vi "Close All Current Shunts.vi"(8 "error in":errorcluster, 11 "Scan Configuration":T2[](array[typedef]) {"Resolution in Digits" items=["3 1/2"=3.5, "4 1/2"=4.5, "5 1/2"=5.5, "6 1/2"=6.5, "7 1/2"=7.5]}) -> (0 "error out":errorcluster, 3 "Array of Shunt to close":T1[](array[typedef]))   [LabVIEW 2021, in "DMM_Scan PXI RLY Driver 32V-16C.lvlib"]
doc: "Uses the scan configuration to return only the current channels and formats them in Individual Switch Relay format."
uses:
  DMM_Scan PXI RLY Driver 32V-16C.lvlib
  Typedefs/Scan configuration.ctl
  <instrlib>/niDMM/nidmm.llb/niDMM Resolution in Digits.ctl
  Static Digital Path Generation/Typedefs/Terminal and State Settings.ctl
  Static Digital Path Generation/Switch_Static Digital Path Generation.lvlib
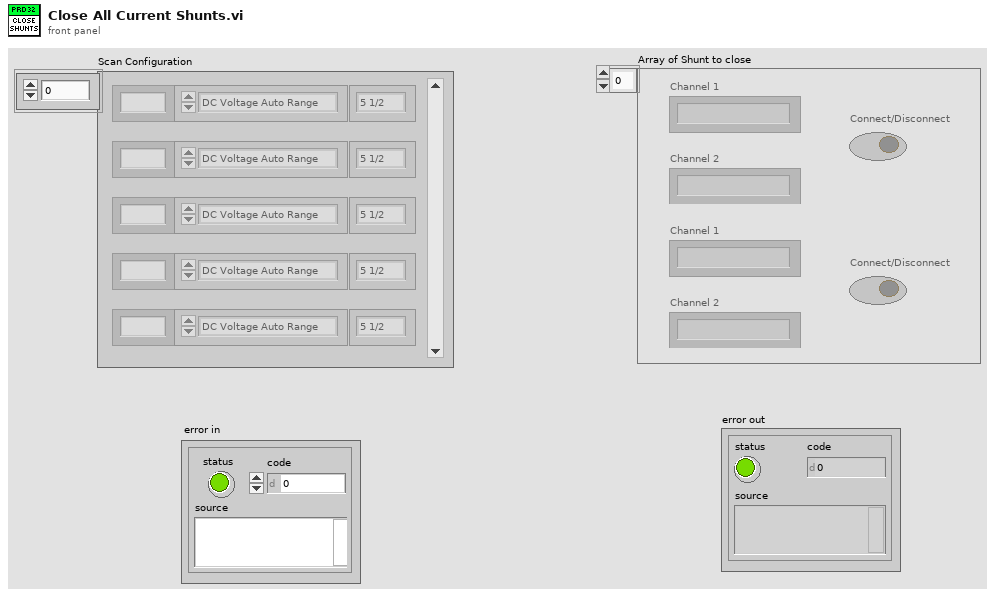
[diagram p1: front panel]
types:
  T1 = typedef "Switch_Static Digital Path Generation.lvlib/Terminal and State Settings.ctl" = cluster{"Connect/Disconnect":bool, "Channel 1":string, "Channel 2":string}
  T2 = typedef "DMM_Scan PXI RLY Driver 32V-16C.lvlib/Scan configuration.ctl" = cluster{"Channel":string, "Resolution in Digits":T3, "Range and Function":enum16{"DC Voltage Auto Range", "DC 100 mV", "DC 1 V ", "DC 10 V", "DC 100 V", "DC 300 V", " ", "AC Voltage Auto Range", "AC 50 mV", "AC 200 mV", "AC 500 mV", "AC 2 V", "AC 5 V", "AC 20 V", "AC 50 V", "AC 300 V", "  ", "DC Current Auto Range", "DC 1 uA", "DC 10 uA", "DC 100 uA", "DC 1 mA", "DC 10 mA", "DC 20 mA", "DC 100 mA", "DC 200 mA", "DC 1 A", "DC 3 A", "   ", "AC Current Auto Range", "AC 100 uA", "AC 1 mA", "AC 10 mA", "AC 100 mA", "AC 500 mA", "AC 1 A", "AC 3 A", "    ", "Resistance Auto Range", "Res 100 Ohm", "Res 1 kOhm", "Res 10 kOhm", "Res 100 kOhm", "Res 1 MOhm", "Res 10 MOhm", "Res 100 MOhm", "Res 5 GOhm", "     ", "Frequency AC Auto Range", "Freq AC 50 mV", "Freq AC 500 mV", "Freq AC 5 V", "Freq AC 50 V", "Freq AC 300 V", "      ", "Period AC Auto Range", "Period AC 50 mV", "Period AC 500 mV", "Period AC 5 V", "Period AC 50 V", "Period AC 300 V"}}
  T3 = typedef "niDMM Resolution in Digits.ctl" = dbl
  T4 = enum16{"DC Voltage Auto Range", "DC 100 mV", "DC 1 V ", "DC 10 V", "DC 100 V", "DC 300 V", " ", "AC Voltage Auto Range", "AC 50 mV", "AC 200 mV", "AC 500 mV", "AC 2 V", "AC 5 V", "AC 20 V", "AC 50 V", "AC 300 V", "  ", "DC Current Auto Range", "DC 1 uA", "DC 10 uA", "DC 100 uA", "DC 1 mA", "DC 10 mA", "DC 20 mA", "DC 100 mA", "DC 200 mA", "DC 1 A", "DC 3 A", "   ", "AC Current Auto Range", "AC 100 uA", "AC 1 mA", "AC 10 mA", "AC 100 mA", "AC 500 mA", "AC 1 A", "AC 3 A", "    ", "Resistance Auto Range", "Res 100 Ohm", "Res 1 kOhm", "Res 10 kOhm", "Res 100 kOhm", "Res 1 MOhm", "Res 10 MOhm", "Res 100 MOhm", "Res 5 GOhm", "     ", "Frequency AC Auto Range", "Freq AC 50 mV", "Freq AC 500 mV", "Freq AC 5 V", "Freq AC 50 V", "Freq AC 300 V", "      ", "Period AC Auto Range", "Period AC 50 mV", "Period AC 500 mV", "Period AC 5 V", "Period AC 50 V", "Period AC 300 V"}
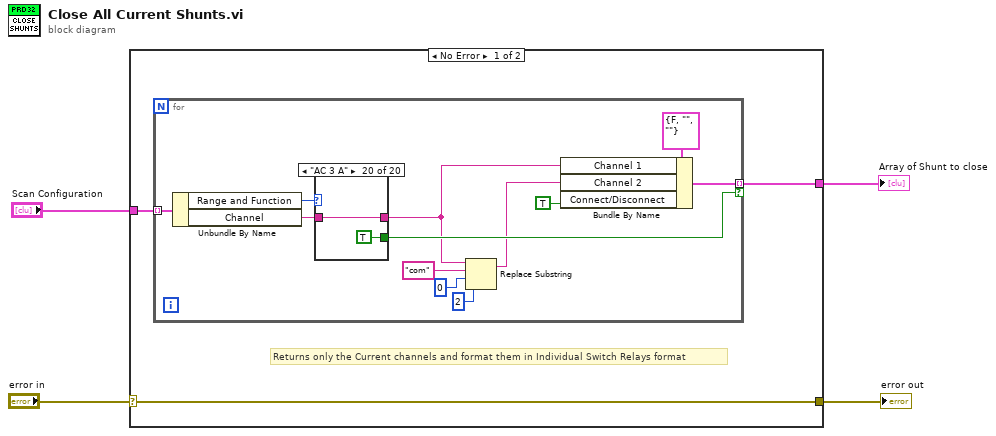
[diagram p0: block diagram]
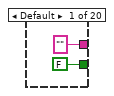
[diagram p2: hidden frame]
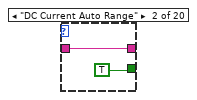
[diagram p3: hidden frame]
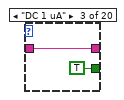
[diagram p4: hidden frame]
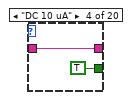
[diagram p5: hidden frame]
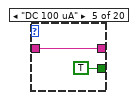
[diagram p6: hidden frame]
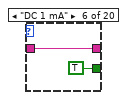
[diagram p7: hidden frame]
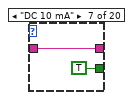
[diagram p8: hidden frame]
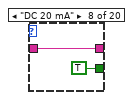
[diagram p9: hidden frame]
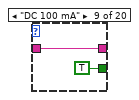
[diagram p10: hidden frame]
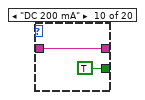
[diagram p11: hidden frame]
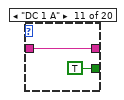
[diagram p12: hidden frame]
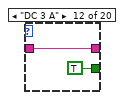
[diagram p13: hidden frame]
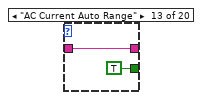
[diagram p14: hidden frame]
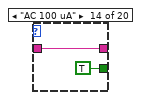
[diagram p15: hidden frame]
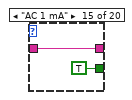
[diagram p16: hidden frame]
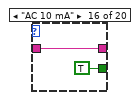
[diagram p17: hidden frame]
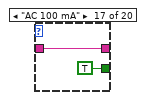
[diagram p18: hidden frame]
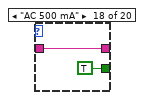
[diagram p19: hidden frame]
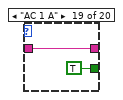
[diagram p20: hidden frame]
diagram:
  n1 = case shown="No Error" "error in" {
    selector: "error in" -> [w5 w61]
    tunnel: "Scan Configuration" -> [w7 _]
    tunnel: [w6 T1[] []] -> w3
    tunnel: [w5 w61] -> w1
    frame No Error {
      # "Returns only the Current channels and format them in Individual Switch Relays format"
      n2 = for {
        tunnel: w7 -> [w19] mode=indexing
        tunnel: [w8] -> w6 mode=indexing if=w13
        n3 = Unbundle By Name(w19) -> ("Range and Function"=w18:T4, "Channel"=w17:string)
        n4 = case shown="\"AC 3 A\"" w18 {
          tunnel: w17 -> [_ w23 w25 w27 w29 w31 w33 w35 w37 w39 w41 w43 w45 w47 w49 w51 w53 w55 w57 w59]
          tunnel: ["" ("Channel") w23 w25 w27 w29 w31 w33 w35 w37 w39 w41 w43 w45 w47 w49 w51 w53 w55 w57 w59] -> w10
          tunnel: [FALSE TRUE TRUE TRUE TRUE TRUE TRUE TRUE TRUE TRUE TRUE TRUE TRUE TRUE TRUE TRUE TRUE TRUE TRUE TRUE] -> w13
          frame Default {
          }
          frame "DC Current Auto Range" {
          }
          frame "DC 1 uA" {
          }
          frame "DC 10 uA" {
          }
          frame "DC 100 uA" {
          }
          frame "DC 1 mA" {
          }
          frame "DC 10 mA" {
          }
          frame "DC 20 mA" {
          }
          frame "DC 100 mA" {
          }
          frame "DC 200 mA" {
          }
          frame "DC 1 A" {
          }
          frame "DC 3 A" {
          }
          frame "AC Current Auto Range" {
          }
          frame "AC 100 uA" {
          }
          frame "AC 1 mA" {
          }
          frame "AC 10 mA" {
          }
          frame "AC 100 mA" {
          }
          frame "AC 500 mA" {
          }
          frame "AC 1 A" {
          }
          frame "AC 3 A" {
          }
        }
        n5 = Replace Substring(2:2 ("length (len. of substring)"), 3:0 ("offset (0)"), 4:"com" ("substring (\"\")"), 5:w10) -> (1:w9:string)  [unwired: 1 out]
        n6 = Bundle By Name(cluster=T1 {"Connect/Disconnect"=FALSE, "Channel 1"="", "Channel 2"=""} ("Terminal and State Settings"), "Channel 1"=w10, "Channel 2"=w9, "Connect/Disconnect"=TRUE) -> (w8:T1)
      }
    }
    frame Error {
    }
  }
  "Array of Shunt to close" <- w3
  "error out" <- w1
